vi "demo.vi"() -> ()   [LabVIEW 2012]
uses:
  type def/Hyde&Show.ctl
  nodos.ctl
  SubVIs/typedef/User Accounts.ctl
panel:
  out "error out":errorcluster
  in  "Read\nUsers":bool
  in  "New\nUser":bool
  in  "Read\nLog":bool
  in  "stop":bool
  out "Out 4":bool
  out "Out 3":bool
  out "Out 2":bool
  out "Out 1":bool
  in  "In 4":bool
  in  "In 3":bool
  in  "In 2":bool
  in  "In 1":bool
  # "Name/Password\nadmin/admin\nuser/user"
  # "Hide for \nusers"
  # "Disabled\nfor user"
  # "grayed for\nusers"
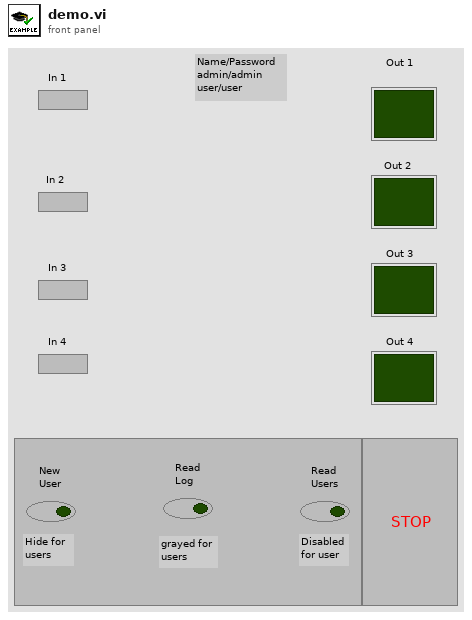
[diagram p1: front panel]
types:
  T1 = typedef "Hyde&Show.ctl" = enum8{"Enabled", "Disabled", " Grayed Out", "Hide"}
  T2 = typedef "nodos.ctl" = enum16{"Default", "Login", "Create", "Running", "Cluse User", "Close Conections", "End"}
  T3 = typedef "User Accounts.ctl" = enum16{"None", "User", "Admin"}
  T4 = typedef "User_Data_Cluster.ctl" = cluster{"Usuario":string, "Password":string, "Account type":T3, "Time Stamp":timestamp}
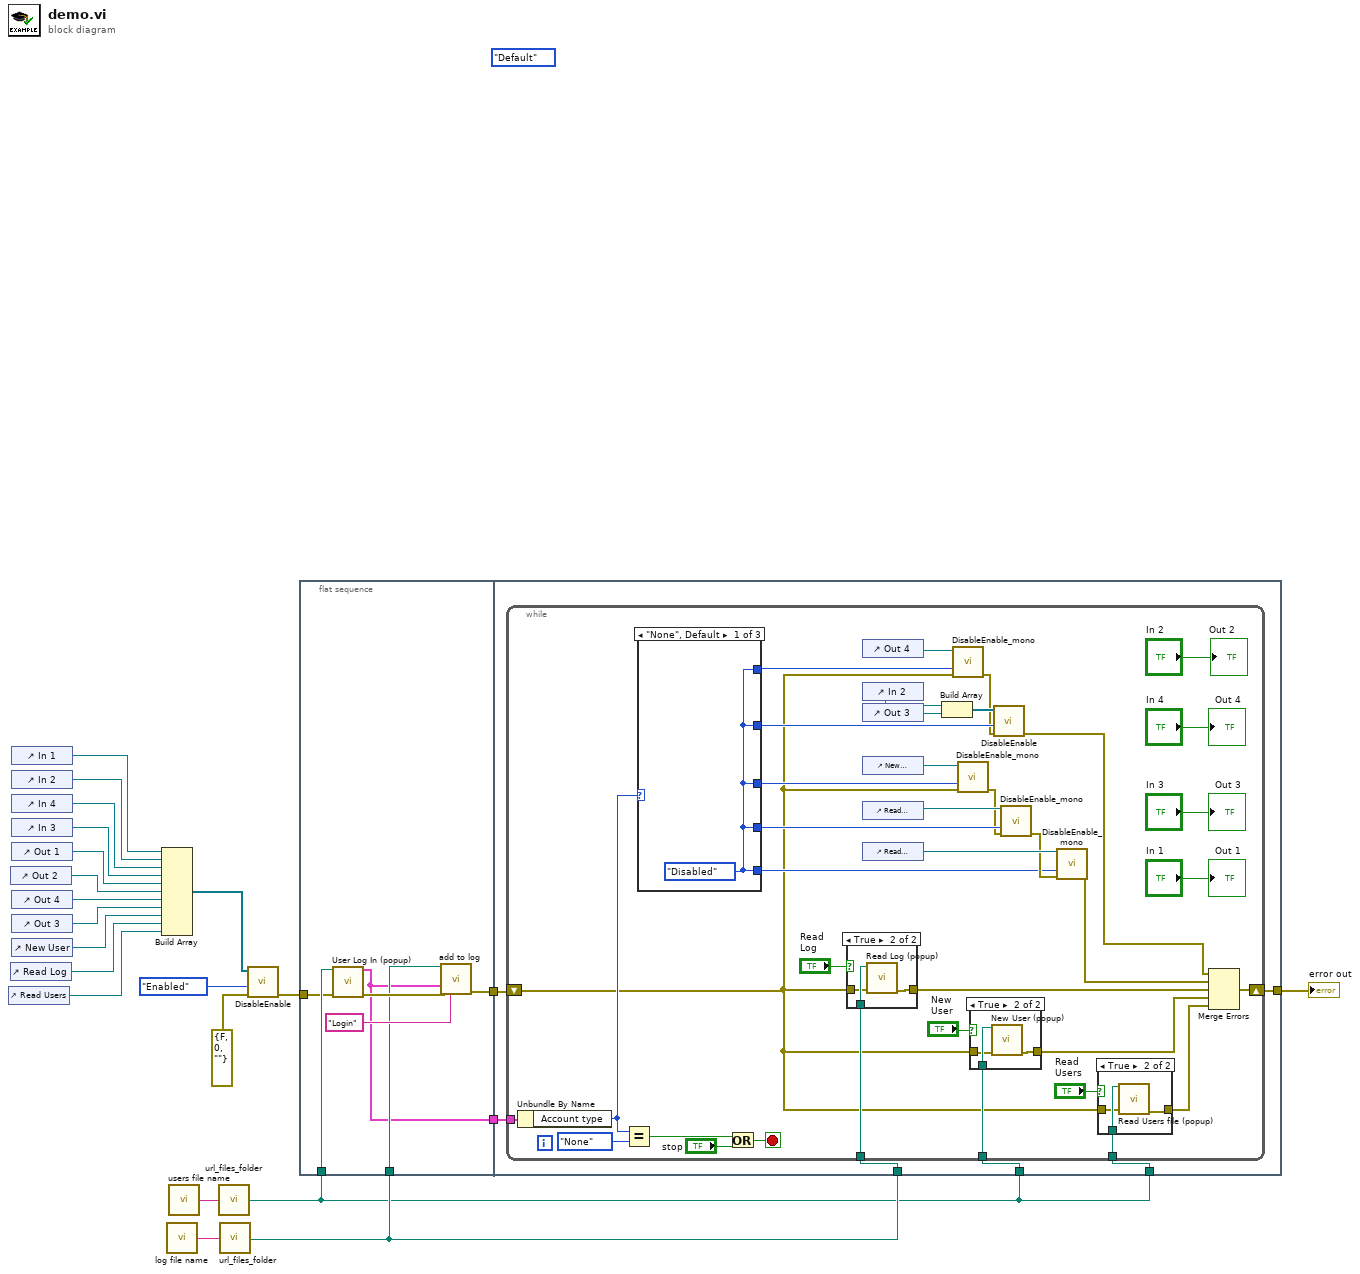
[diagram p0: block diagram]
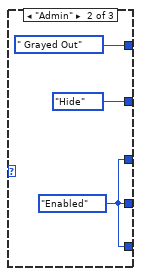
[diagram p5: hidden frame]
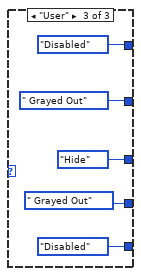
[diagram p6: hidden frame]
diagram:
  (unwired) nodos."Default"
  n1 = control-ref of="Read Users"() -> (w4:refnum<vi>)
  n2 = control-ref of="Out 2"() -> (w8:refnum<vi>)
  n3 = control-ref of="Read Log"() -> (w2:refnum<vi>)
  n4 = control-ref of="In 1"() -> (w13:refnum<vi>)
  n5 = control-ref of="In 2"() -> (w12:refnum<vi>)
  n6 = control-ref of="In 4"() -> (w11:refnum<vi>)
  n7 = control-ref of="In 3"() -> (w10:refnum<vi>)
  n8 = control-ref of="Out 1"() -> (w9:refnum<vi>)
  n9 = control-ref of="Out 4"() -> (w7:refnum<vi>)
  n10 = control-ref of="Out 3"() -> (w6:refnum<vi>)
  n11 = control-ref of="New User"() -> (w5:refnum<vi>)
  n12 = Build Array(w13, w12, w11, w10, w9, w8, w7, w6, w5, w2, w4) -> (w3:refnum<vi>[])
  n13 = call "log file name.vi"() -> ("file name"=w21:string)  [unwired: 15 in]
  n14 = call "users file name.vi"() -> ("file name"=w22:string)  [unwired: 15 in]
  n15 = call "url_files_folder.vi"("file name"=w22) -> ("Path"=w18:path)  [unwired: 14 in]
  n16 = call "url_files_folder.vi"("file name"=w21) -> ("Path"=w19:path)  [unwired: 14 in]
  n17 = call "DisableEnable.vi"("error in (no error)"=errorcluster {"status"=FALSE, "code"=0, "source"=""} ("error constant"), "Action 2"=Hyde&Show."Enabled", "Array of Control References"=w3) -> ("error out"=w16:errorcluster)  [unwired: 8 in]
  n18 = flat-sequence {
    tunnel: w18 -> [w27]
    tunnel: w19 -> [w26]
    tunnel: [w25] -> w20
    tunnel: [w24] -> w17
    tunnel: w16 -> [w23]
    tunnel: w20 -> [w35]
    tunnel: w19 -> [w34]
    tunnel: w18 -> [w33]
    tunnel: w18 -> [w32]
    tunnel: w17 -> [w31]
    tunnel: [w30] -> w1
    frame #0 {
      n19 = call "User Log In (popup).vi"(0:w27, "error in (no error)"=w23) -> ("User-data cluster Out"=w25:T4, "error out"=w29:errorcluster)  [unwired: 11 in, 1 out]
      n20 = call "add to log.vi"("Path"=w26, "User-data cluster"=w25, "error in (no error)"=w29, "Data"="Login") -> ("error out"=w24:errorcluster)  [unwired: 11 in]
    }
    frame #1 {
      n21 = while {
        tunnel: w35 -> [w66]
        tunnel: w34 -> [w60]
        tunnel: w33 -> [w59]
        tunnel: w32 -> [w58]
        shift-right: [w57] -> w30
        shift-left: w31 -> [w37]
        stop <- w72 stop-if-true
        n22 = Unbundle By Name(w66) -> ("Account type"=w49:T3)
        n23 = Equal?(x=w49, y=User_Accounts."None") -> (x = y?=w70:bool)
        n24 = case shown="\"None\", Default" w49 {
          tunnel: [w86 w89 Hyde&Show."Hide" ("Action 2")] -> w62
          tunnel: [w86 w89 Hyde&Show." Grayed Out" ("Action 2")] -> w61
          tunnel: [w86 w89 Hyde&Show."Disabled" ("Action 2")] -> w50
          tunnel: [w86 Hyde&Show." Grayed Out" ("Action 2") Hyde&Show."Disabled" ("Action 2")] -> w41
          tunnel: [w86 Hyde&Show."Hide" ("Action 2") Hyde&Show." Grayed Out" ("Action 2")] -> w42
          frame "None", Default {
            w86 = Hyde&Show."Disabled" ("Action 2")
          }
          frame "Admin" {
            w89 = Hyde&Show."Enabled" ("Action 2")
          }
          frame "User" {
          }
        }
        n25 = Or(x=w70, y="stop") -> (x .or. y?=w72:bool)
        n26 = case shown="True" "Read\nLog" {
          tunnel: w60 -> [_ w81]
          tunnel: [w78 w80] -> w55
          tunnel: w37 -> [w78 w79]
          frame False {
          }
          frame True {
            n27 = call "Read Log (popup).vi"("error in (no error)"=w79, "file path (use dialog)"=w81) -> ("error out"=w80:errorcluster)  [unwired: 9 in]
          }
        }
        n28 = control-ref of="Out 4"() -> (w40:refnum<vi>)
        n29 = control-ref of="In 2"() -> (w36:refnum<vi>)
        n30 = control-ref of="Out 3"() -> (w43:refnum<vi>)
        n31 = control-ref of="New\nUser"() -> (w63:refnum<vi>)
        n32 = control-ref of="Read\nLog"() -> (w65:refnum<vi>)
        n33 = control-ref of="Read\nUsers"() -> (w64:refnum<vi>)
        n34 = Build Array(w36, w43) -> (w44:refnum<vi>[])
        n35 = call "DisableEnable_mono.vi"("Control in"=w40, "Action in"=w41, "error in (no error)"=w37) -> ("error out"=w38:errorcluster)  [unwired: 12 in]
        n36 = call "DisableEnable_mono.vi"("Control in"=w63, "Action in"=w62, "error in (no error)"=w37) -> ("error out"=w53:errorcluster)  [unwired: 12 in]
        n37 = case shown="True" "New\nUser" {
          tunnel: w59 -> [_ w85]
          tunnel: [w82 w84] -> w54
          tunnel: w37 -> [w82 w83]
          frame False {
          }
          frame True {
            n38 = call "New User (popup).vi"("file path (use dialog)"=w85, "error in (no error)"=w83) -> ("error out"=w84:errorcluster)  [unwired: 13 in]
          }
        }
        n39 = call "DisableEnable.vi"("error in (no error)"=w38, "Action 2"=w42, "Array of Control References"=w44) -> ("error out"=w39:errorcluster)  [unwired: 8 in]
        n40 = call "DisableEnable_mono.vi"("Control in"=w65, "Action in"=w61, "error in (no error)"=w53) -> ("error out"=w52:errorcluster)  [unwired: 12 in]
        n41 = call "DisableEnable_mono.vi"("Control in"=w64, "Action in"=w50, "error in (no error)"=w52) -> ("error out"=w51:errorcluster)  [unwired: 12 in]
        n42 = case shown="True" "Read\nUsers" {
          tunnel: w58 -> [_ w77]
          tunnel: [w74 w76] -> w56
          tunnel: w37 -> [w74 w75]
          frame False {
          }
          frame True {
            n43 = call "Read Users file (popup).vi"("file path (use dialog)"=w77, "error in (no error)"=w75) -> ("error out"=w76:errorcluster)  [unwired: 13 in]
          }
        }
        n44 = Merge Errors(w39, w51, w55, w54, w56) -> (w57:errorcluster)
        "Out 1" <- "In 1"
        "Out 2" <- "In 2"
        "Out 3" <- "In 3"
        "Out 4" <- "In 4"
      }
    }
  }
  "error out" <- w1
